vi "PNEU_Write_Refnum.vi"(7 "Shooter_Arm":T5, 8 "Flipper":T5, 9 "Gear":T5, 10 "Intake_Arm":T5, 11 "Pneu":T1) -> ()   [LabVIEW 2015]
uses:
  <vilib>/Rock Robotics/WPI/Solenoid/WPI_SolenoidValue.ctl
  Ref_Num/Pneu_Type_Def.ctl
  <vilib>/Rock Robotics/WPI/Solenoid/WPI_SolenoidDevRef.ctl
  <vilib>/Rock Robotics/WPI/Solenoid/WPI_SolenoidChannel.ctl
  <vilib>/Rock Robotics/WPI/Compressor/WPI_CompressorDevRef.ctl
  <vilib>/Rock Robotics/WPI/Solenoid/WPI_SolenoidSetEnum.vi
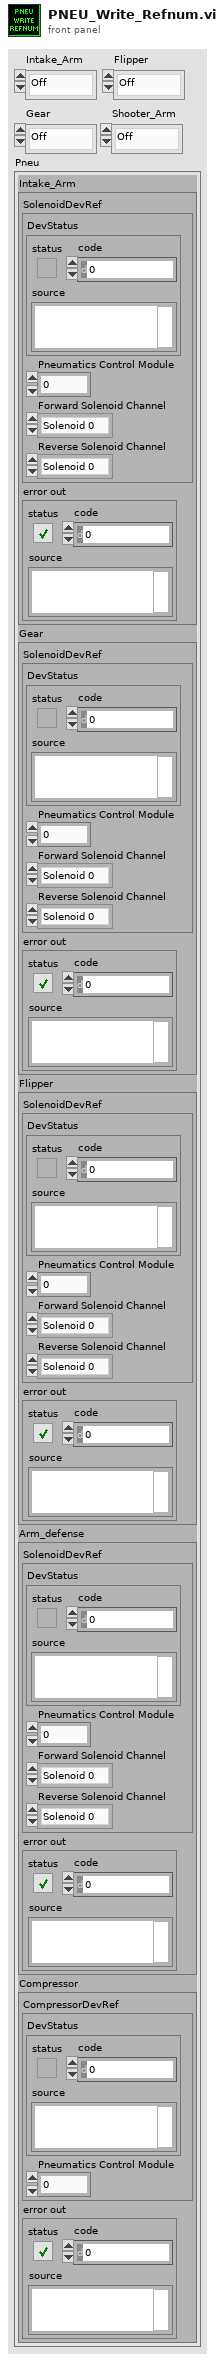
[diagram p1: front panel]
types:
  T1 = typedef "Pneu_Type_Def.ctl" = cluster{"Intake_Arm":cluster{"SolenoidDevRef":T2, "error out":errorcluster}, "Gear":cluster{"SolenoidDevRef":T2, "error out":errorcluster}, "Flipper":cluster{"SolenoidDevRef":T2, "error out":errorcluster}, "Arm_defense":cluster{"SolenoidDevRef":T2, "error out":errorcluster}, "Compressor":cluster{"CompressorDevRef":T4, "error out":errorcluster}}
  T2 = typedef "WPI_SolenoidDevRef.ctl" = cluster{"DevStatus":errorcluster, "Pneumatics Control Module":u8, "Forward Solenoid Channel":T3, "Reverse Solenoid Channel":T3}
  T3 = typedef "WPI_SolenoidChannel.ctl" = enum8{"Solenoid 0", "Solenoid 1", "Solenoid 2", "Solenoid 3", "Solenoid 4", "Solenoid 5", "Solenoid 6", "Solenoid 7", "Invalid"}
  T4 = typedef "WPI_CompressorDevRef.ctl" = cluster{"DevStatus":errorcluster, "Pneumatics Control Module":u8}
  T5 = typedef "WPI_SolenoidValue.ctl" = enum16{"Off", "On", "Forward", "Reverse"}
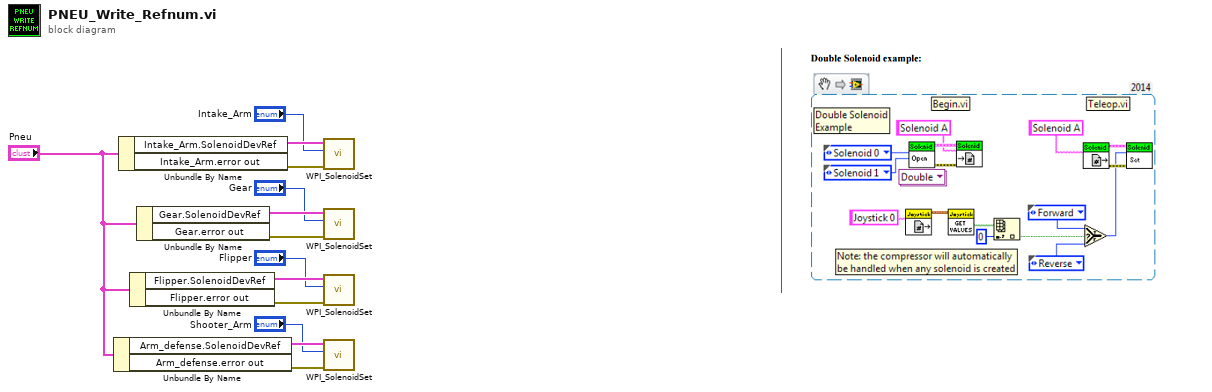
[diagram p0: block diagram]
diagram:
  n1 = Unbundle By Name("Pneu") -> ("Arm_defense.SolenoidDevRef"=w6:T2, "Arm_defense.error out"=w7:errorcluster)
  n2 = Unbundle By Name("Pneu") -> ("Intake_Arm.SolenoidDevRef"=w13:T2, "Intake_Arm.error out"=w12:errorcluster)
  n3 = Unbundle By Name("Pneu") -> ("Flipper.SolenoidDevRef"=w9:T2, "Flipper.error out"=w8:errorcluster)
  n4 = Unbundle By Name("Pneu") -> ("Gear.SolenoidDevRef"=w10:T2, "Gear.error out"=w11:errorcluster)
  n5 = call-poly <vilib>:"WPI_SolenoidSet.vi"("error in (no error)"=w12, "Value"="Intake_Arm", "SolenoidDevRef"=w13) -> ()  [unwired: 7 in, 2 out]
  n6 = call-poly <vilib>:"WPI_SolenoidSet.vi"("error in (no error)"=w11, "Value"="Gear", "SolenoidDevRef"=w10) -> ()  [unwired: 7 in, 2 out]
  n7 = call-poly <vilib>:"WPI_SolenoidSet.vi"("error in (no error)"=w8, "Value"="Flipper", "SolenoidDevRef"=w9) -> ()  [unwired: 7 in, 2 out]
  n8 = call-poly <vilib>:"WPI_SolenoidSet.vi"("error in (no error)"=w7, "Value"="Shooter_Arm", "SolenoidDevRef"=w6) -> ()  [unwired: 7 in, 2 out]
